vi "Read SwitchDMM Channel.vi"(8 "error in (no error)":errorcluster, 11 "DMM Channel configuration":refnum<class "SwitchDMM Channel configuration.lvclass">) -> (0 "error out":errorcluster, 2 "SwitchDMM Channel":T1={"Switch"="Switch0"}, 3 "DMM Channel configuration out":refnum<class "SwitchDMM Channel configuration.lvclass">)   [LabVIEW 2025, in "SwitchDMM Channel configuration.lvclass"]
uses:
  SwitchDMM Channel configuration.lvclass
  SwitchDMM Channel.ctl
  SwitchDMM Channel configuration.lvclass/SwitchDMM Channel configuration.ctl
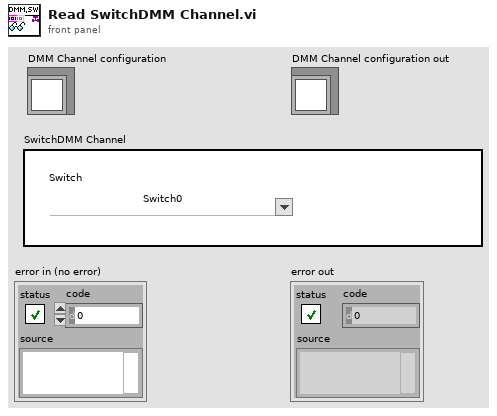
[diagram p1: front panel]
types:
  T1 = typedef "SwitchDMM Channel configuration.lvclass/SwitchDMM Channel.ctl" = cluster{"Switch":string}
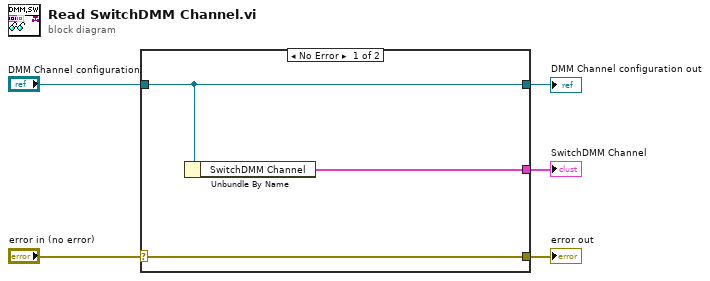
[diagram p0: block diagram]
diagram:
  n1 = case shown="No Error" "error in (no error)" {
    selector: "error in (no error)" -> [w8 w9]
    tunnel: [w8 w9] -> w4
    tunnel: [w7 w10] -> w3
    tunnel: "DMM Channel configuration" -> [w7 w10]
    tunnel: [w6 _] -> w1
    frame No Error {
      n2 = Unbundle By Name(w7) -> ("SwitchDMM Channel"=w6:T1)
    }
    frame Error {
    }
  }
  "error out" <- w4
  "DMM Channel configuration out" <- w3
  "SwitchDMM Channel" <- w1
